vi "Write Array of Sequences.vi"(8 "error in (no error)":errorcluster, 10 "Array of Seqs":refnum<class "Sequence of SBlocks.lvclass">[](array[class]), 11 "Scheduler in":refnum<class "Scheduler.lvclass">=refnum) -> (0 "error out":errorcluster, 3 "Scheduler out":refnum<class "Scheduler.lvclass">)   [LabVIEW 2020, in "CIRCUS_uServices.lvlib" / "Scheduler.lvlib" / "Scheduler.lvclass"]
uses:
  Scheduler.lvclass
  Scheduler.lvclass/Scheduler.ctl
  Run Utilities/Sequence of SBlocks/Sequence of SBlocks.lvclass
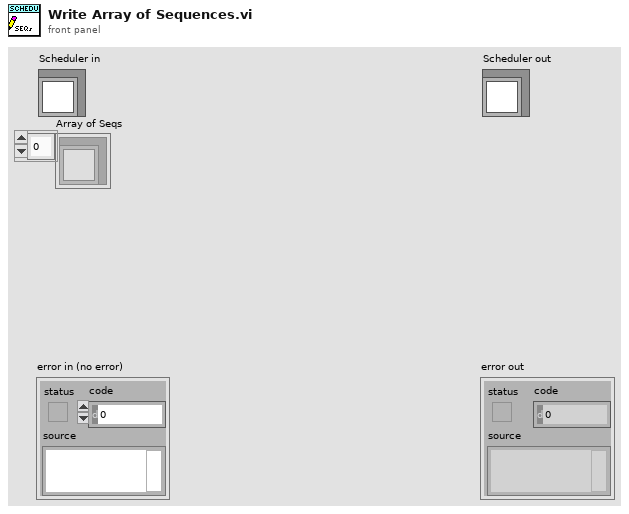
[diagram p1: front panel]
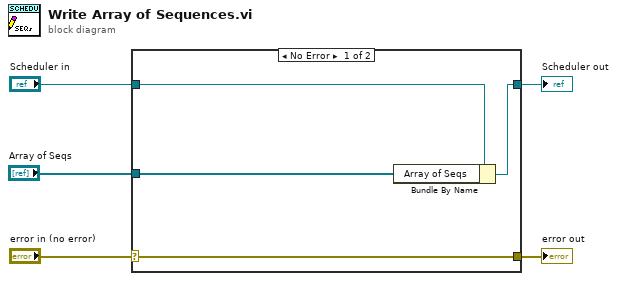
[diagram p0: block diagram]
diagram:
  n1 = case shown="No Error" "error in (no error)" {
    selector: "error in (no error)" -> [w9 w10]
    tunnel: [w9 w10] -> w4
    tunnel: [w7 w11] -> w2
    tunnel: "Scheduler in" -> [w8 w11]
    tunnel: "Array of Seqs" -> [w6 _]
    frame No Error {
      n2 = Bundle By Name(cluster=w8, "Array of Seqs"=w6) -> (w7:refnum<class "Scheduler.lvclass">)
    }
    frame Error {
    }
  }
  "error out" <- w4
  "Scheduler out" <- w2
